vi "testStopServersAandBMultipleTimes.vi"(8 "error in (no error)":errorcluster) -> (0 "error out":errorcluster)   [LabVIEW 2018]
uses:
  <vilib>/addons/_JKI Toolkits/Caraya/classes/Test/Test.lvclass
  <vilib>/addons/_JKI Toolkits/Caraya/classes/Assert/Assert.lvclass
  <vilib>/addons/_JKI Toolkits/Caraya/classes/Assert/Assert Equal Value_Variant.vi
  src/FactoryTcpServer/FactoryTcpServer.lvclass
  src/TcpServer/TcpServer.lvclass
  src/TcpServerBase/TcpServerBase.lvclass
  src/TcpServerCmd/TcpServerCmd.lvclass
  home/pcortes/Documents/github/ts_labview_tcp_json/src/TcpServerBase/TcpServerBase.lvclass
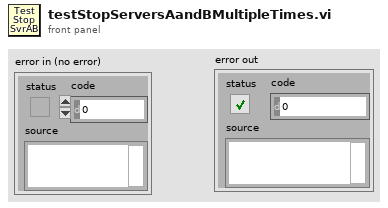
[diagram p1: front panel]
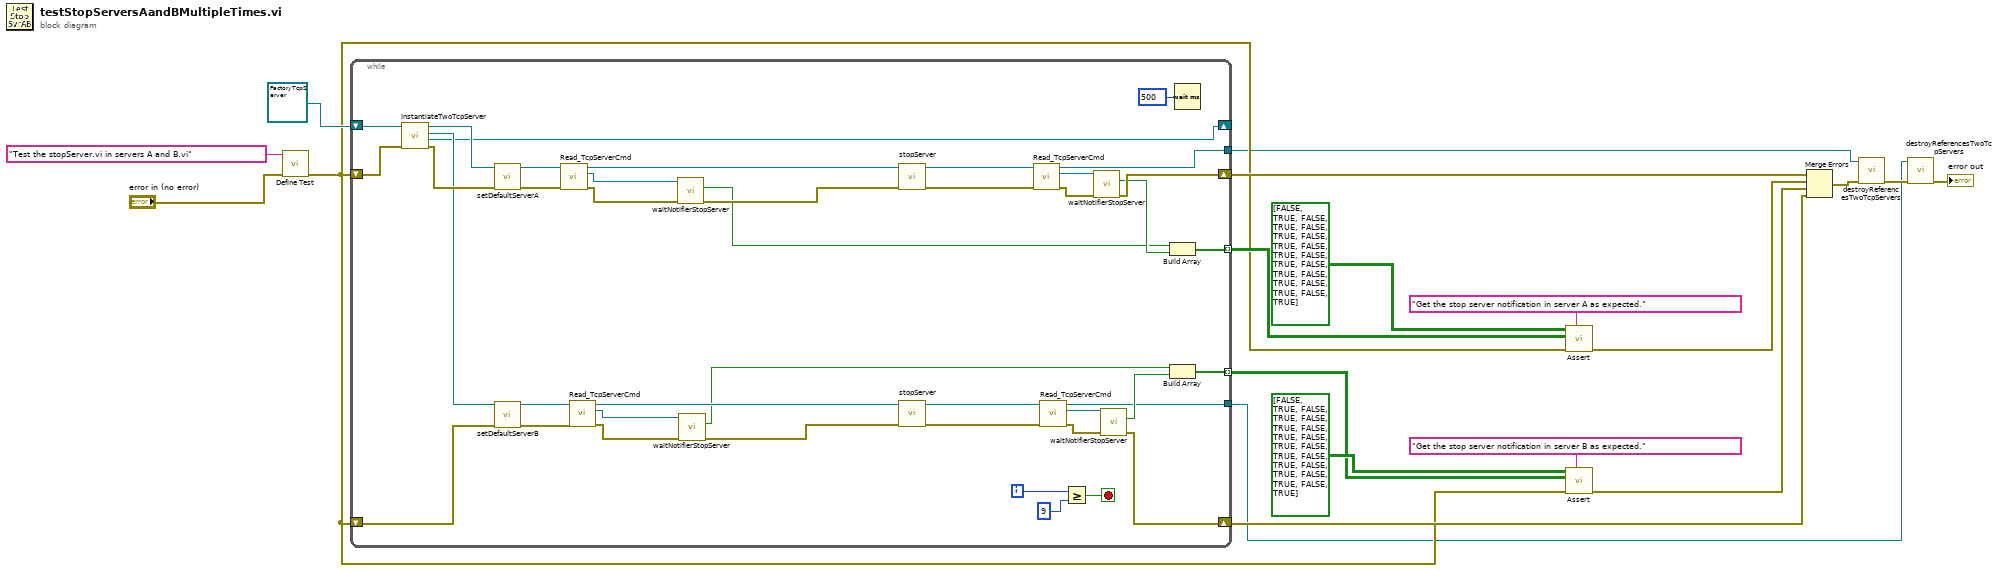
[diagram p0: block diagram]
diagram:
  n1 = call <vilib>:"Define Test.vi"("error in (no error)"="error in (no error)", "Label (VI Title)"="Test the stopServer.vi in servers A and B.vi") -> ("error out"=w5:errorcluster)  [unwired: 9 in]
  n2 = while {
    shift-right: [w58] -> w16
    shift-left: w5 -> [w27]
    tunnel: [w30] -> w10 mode=indexing
    tunnel: [w29] -> w7 mode=indexing
    shift-right: [w23] -> _
    shift-left: refnum<class "FactoryTcpServer.lvclass"> refnum ("FactoryTcpServer in") -> [w28]
    shift-right: [w48] -> w11
    shift-left: w5 -> [w22]
    tunnel: [w21] -> w3
    tunnel: [w20] -> w1
    i -> [w33]
    stop <- w31 stop-if-true
    n3 = call "instantiateTwoTcpServer.vi"("error in (no error)"=w27, "FactoryTcpServer in"=w28) -> ("error out"=w25:errorcluster, "FactoryTcpServer out"=w23:refnum<class "FactoryTcpServer.lvclass">, "TcpServer 2 out"=w24:refnum<class "TcpServer.lvclass">, "TcpServer 1 out"=w26:refnum<class "TcpServer.lvclass">)  [unwired: 6 in]
    n4 = call "setDefaultServerA.vi"("error in (no error)"=w25, "TcpServer.lvclass"=w26) -> ("error out"=w52:errorcluster, "tcpServer out"=w53:refnum<class "TcpServer.lvclass">)  [unwired: 8 in]
    n5 = call "setDefaultServerB.vi"("error in (no error)"=w22, "TcpServer.lvclass"=w24) -> ("error out"=w44:errorcluster, "tcpServer out"=w45:refnum<class "TcpServer.lvclass">)  [unwired: 8 in]
    n6 = call "Read_TcpServerCmd.vi"("error in (no error)"=w52, "TcpServer in"=w53) -> ("error out"=w37:errorcluster, "TcpServerCmd.lvclass"=w36:refnum<class "TcpServerCmd.lvclass">, "TcpServer out"=w60:refnum<class "TcpServer.lvclass">)  [unwired: 7 in]
    n7 = call "Read_TcpServerCmd.vi"("error in (no error)"=w44, "TcpServer in"=w45) -> ("error out"=w38:errorcluster, "TcpServerCmd.lvclass"=w35:refnum<class "TcpServerCmd.lvclass">, "TcpServer out"=w46:refnum<class "TcpServer.lvclass">)  [unwired: 7 in]
    n8 = call "waitNotifierStopServer.vi"("error in (no error)"=w37, "TcpServerBase in"=w36) -> ("error out"=w59:errorcluster, "stopServer"=w41:bool)  [unwired: 7 in, 1 out]
    n9 = call "waitNotifierStopServer.vi"("error in (no error)"=w38, "TcpServerBase in"=w35) -> ("error out"=w47:errorcluster, "stopServer"=w34:bool)  [unwired: 7 in, 1 out]
    n10 = call "stopServer.vi"("error in (no error)"=w59, "tcpServer in"=w60) -> ("error out"=w56:errorcluster, "tcpServer out"=w57:refnum<class "TcpServer.lvclass">)  [unwired: 8 in]
    n11 = call "stopServer.vi"("error in (no error)"=w47, "tcpServer in"=w46) -> ("error out"=w42:errorcluster, "tcpServer out"=w43:refnum<class "TcpServer.lvclass">)  [unwired: 8 in]
    n12 = call "Read_TcpServerCmd.vi"("error in (no error)"=w56, "TcpServer in"=w57) -> ("error out"=w54:errorcluster, "TcpServerCmd.lvclass"=w55:refnum<class "TcpServerCmd.lvclass">, "TcpServer out"=w21:refnum<class "TcpServer.lvclass">)  [unwired: 7 in]
    n13 = call "Read_TcpServerCmd.vi"("error in (no error)"=w42, "TcpServer in"=w43) -> ("error out"=w50:errorcluster, "TcpServerCmd.lvclass"=w49:refnum<class "TcpServerCmd.lvclass">, "TcpServer out"=w20:refnum<class "TcpServer.lvclass">)  [unwired: 7 in]
    n14 = Greater Or Equal?(x=w33, y=9) -> (x >= y?=w31:bool)
    n15 = call "waitNotifierStopServer.vi"("error in (no error)"=w54, "TcpServerBase in"=w55) -> ("error out"=w58:errorcluster, "stopServer"=w51:bool)  [unwired: 7 in, 1 out]
    n16 = call "waitNotifierStopServer.vi"("error in (no error)"=w50, "TcpServerBase in"=w49) -> ("error out"=w48:errorcluster, "stopServer"=w40:bool)  [unwired: 7 in, 1 out]
    n17 = Build Array(w41, w51) -> (w30:bool[])
    n18 = Build Array(w34, w40) -> (w29:bool[])
    n19 = Wait (ms)(milliseconds to wait=u32 500) -> ()  [unwired: 1 out]
  }
  n20 = call-poly <vilib>:"Assert.vi"("Label"="Get the stop server notification in server A as expected.", "error in (no error)"=w5, "Y"=w10, "X"=bool[][] [[FALSE, TRUE], [FALSE, TRUE], [FALSE, TRUE], [FALSE, TRUE], [FALSE, TRUE], [FALSE, TRUE], [FALSE, TRUE], [FALSE, TRUE], [FALSE, TRUE], [FALSE, TRUE]] ("Array 3")) -> ("error out"=w14:errorcluster)  [unwired: 7 in]
  n21 = call-poly <vilib>:"Assert.vi"("Label"="Get the stop server notification in server B as expected.", "error in (no error)"=w5, "Y"=w7, "X"=bool[][] [[FALSE, TRUE], [FALSE, TRUE], [FALSE, TRUE], [FALSE, TRUE], [FALSE, TRUE], [FALSE, TRUE], [FALSE, TRUE], [FALSE, TRUE], [FALSE, TRUE], [FALSE, TRUE]] ("Array 3")) -> ("error out"=w12:errorcluster)  [unwired: 7 in]
  n22 = Merge Errors(w16, w14, w12, w11) -> (w17:errorcluster)
  n23 = call "destroyReferencesTwoTcpServers.vi"("error in (no error)"=w17, "TcpServer in"=w3) -> ("error out"=w4:errorcluster)  [unwired: 8 in, 1 out]
  n24 = call "destroyReferencesTwoTcpServers.vi"("error in (no error)"=w4, "TcpServer in"=w1) -> ("error out"=→"error out":errorcluster)  [unwired: 8 in, 1 out]
